vi "write_and_wait_for_Ackvi.vi"(2 "request":string, 4 "string in front":string, 5 "Operation":string, 6 "error in (no error)":errorcluster, 7 "response":string, 8 "Timeout [ms]":u32=5000, 9 "VISA resource name":refnum<visa-resource-name>) -> (0 "error out":errorcluster, 1 "result":string, 3 "VISA resource name out":refnum<visa-resource-name>)   [LabVIEW 2013]
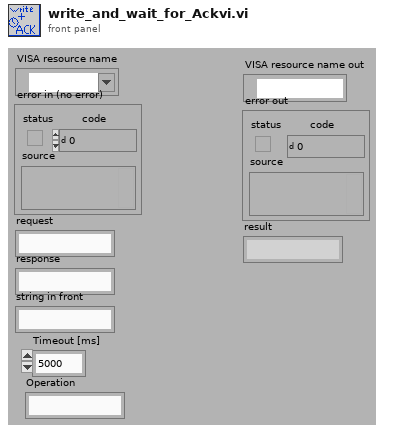
[diagram p1: front panel]
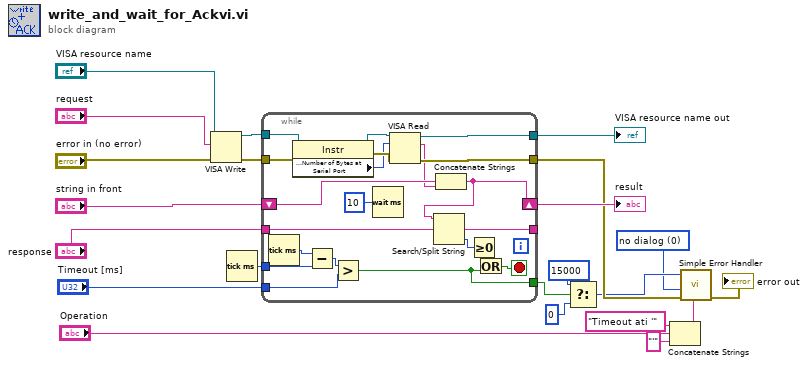
[diagram p0: block diagram]
diagram:
  w1 = u16 0 items=["no dialog", "OK message", "continue or stop message"] ("type of dialog (OK msg:1)")
  n1 = VISA Write(VISA resource name="VISA resource name", write buffer="request", error in (no error)="error in (no error)") -> (VISA resource name out=w22:refnum<visa-resource-name>, error out=w21:errorcluster)  [unwired: 1 out]
  n2 = Tick Count (ms)() -> (millisecond timer value=w13:u32)
  n3 = while {
    tunnel: w21 -> [w35]
    shift-left: "string in front" -> [w41]
    shift-right: [w39] -> w14
    tunnel: [w42] -> w11
    tunnel: [w43] -> w20
    tunnel: w22 -> [w37]
    tunnel: "response" -> [w32]
    tunnel: [w31] -> _
    tunnel: w13 -> [w28]
    tunnel: "Timeout [ms]" -> [w26]
    tunnel: [w23] -> w6
    stop <- w24 stop-if-true
    n4 = Tick Count (ms)() -> (millisecond timer value=w29:u32)
    n5 = property class="Instr"(reference=w37, error in=w35) -> (reference out=w36:refnum<visa-resource-name>, error out=w34:errorcluster, "Serial Settings:Number of Bytes at Serial Port"=w33:u32)
    n6 = Subtract(x=w29, y=w28) -> (x-y=w27:u32)
    n7 = Greater?(x=w27, y=w26) -> (0:w23:bool)
    n8 = Wait (ms)(milliseconds to wait=u32 10) -> ()  [unwired: 1 out]
    n9 = VISA Read(VISA resource name=w36, byte count=w33, error in (no error)=w34) -> (VISA resource name out=w43:refnum<visa-resource-name>, read buffer=w40:string, error out=w42:errorcluster)  [unwired: 1 out]
    n10 = Concatenate Strings(w41, w40) -> (w39:string)
    n11 = Search/Split String(string=w39, search string/char (-)=w32) -> (match + rest of string=w31:string, offset of match=w38:i32)  [unwired: 1 in, 1 out]
    n12 = Greater Or Equal To 0?(x=w38) -> (x >= 0?=w25:bool)
    n13 = Or(x=w25, y=w23) -> (x .or. y?=w24:bool)
  }
  "VISA resource name out" <- w20
  "result" <- w14
  n14 = Select(t=15000, s=w6, f=0) -> (s? t:f=w3:i32)
  n15 = Concatenate Strings("Timeout ati '", "Operation", "'" ("string")) -> (w7:string)
  n16 = call <vilib>:"Simple Error Handler.vi"("error code (no error:0)"=w3, "error source (\" \")"=w7, "type of dialog (OK msg:1)"=w1, "error in (no error)"=w11) -> ("error out"=→"error out":errorcluster)  [unwired: 1 in, 4 out]
